vi "Do.vi"(8 "error in (no error)":errorcluster, 10 "Actor in":refnum<class "Actor.lvclass">, 11 "Analog Input Waveform Data Msg":refnum<class "Analog Input Waveform Data Msg.lvclass">) -> (0 "error out":errorcluster, 2 "Actor out":refnum<class "Actor.lvclass">)   [LabVIEW 2024, in "DAQmx Actor Interface.lvlib" / "Analog Input Waveform Data Msg.lvclass"]
doc: "This VI delivers the message to the actor by calling the appropriate method(s) on the actor."
uses:
  Analog Input Waveform Data Msg.lvclass
  <vilib>/ActorFramework/Actor/Actor.lvclass
  Analog Input Waveform Data Msg.lvclass/Analog Input Waveform Data Msg.ctl
  Analog Input Waveform Data/Analog Input Waveform Data.lvclass
  9ef47adc-f318-494c-9b8b-6df3216d6863.vi
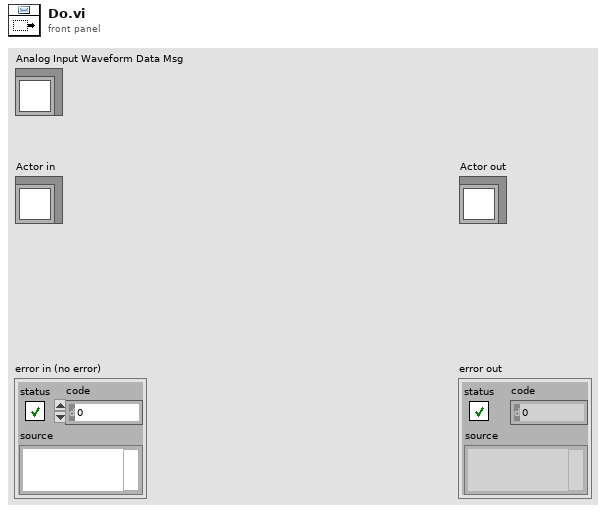
[diagram p1: front panel]
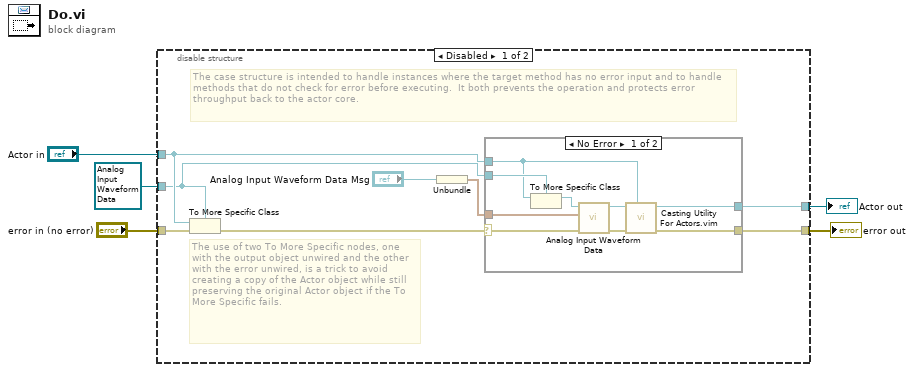
[diagram p0: block diagram]
diagram:
  n1 = disable-structure shown="Disabled" {
    disable-tunnel: "error in (no error)" -> [w12 w25]
    disable-tunnel: [w10 w25] -> w4
    disable-tunnel: [w9 w26] -> w3
    disable-tunnel: "Actor in" -> [w8 w26]
    disable-tunnel: refnum<class "Analog Input Waveform Data.lvclass"> refnum ("Actor in") -> [w7 _]
    frame Disabled {
      # "The use of two To More Specific nodes, one with the output object unwired and the other with the error unwired, is a trick to avoid creating a copy of the Actor object while still preserving the original Actor object if the To More Specific fails."
      # "The case structure is intended to handle instances where the target method has no error input and to handle methods that do not check for error before executing.  It both prevents the operation and protects error throughput back to the actor core."
      n2 = To More Specific Class(target class=w7, reference=w8, error in=w12) -> (error out=w11:errorcluster)  [unwired: 1 out]
      n3 = Unbundle("Analog Input Waveform Data Msg") -> (w6:waveform(dbl)[])
      n4 = case shown="No Error" w11 {
        selector: w11 -> [w22 w24]
        tunnel: [w16 w24] -> w10
        tunnel: [w17 w23] -> w9
        tunnel: w8 -> [w19 w23]
        tunnel: w7 -> [w20 _]
        tunnel: w6 -> [w14 _]
        frame No Error {
          n5 = To More Specific Class(target class=w20, reference=w19) -> (specific class reference=w21:refnum<class "Analog Input Waveform Data.lvclass">)  [unwired: 1 in, 1 out]
          n6 = call-dynamic "Analog Input Waveform Data.vi"("error in (no error)"=w22, "Analog Data"=w14, "Analog Input Waveform Data in"=w21) -> ("error out"=w15:errorcluster, "Analog Input Waveform Data out"=w18:refnum<class "Analog Input Waveform Data.lvclass">)  [unwired: 7 in]
          n7 = call "Casting Utility For Actors.vim"("type"=w19, "error in (no error)"=w15, "Actor in"=w18) -> ("error out"=w16:errorcluster, "Actor out"=w17:refnum<class "Actor.lvclass">)  [unwired: 7 in]
        }
        frame Error {
          # "If type check fails, pass the original object out again."
        }
      }
    }
    frame Enabled {
    }
  }
  "error out" <- w4
  "Actor out" <- w3
